vi "Get Buffer Filling Mode.vi"(0 "VISA resource name":refnum<visa-resource-name>, 5 "Buffer Name (defbuffer1)":string="defbuffer1", 11 "error in (no error)":errorcluster) -> (4 "VISA resource name out":refnum<visa-resource-name>, 6 "Data out":string, 15 "error out":errorcluster)   [LabVIEW 2020, in "Keithley 2450.lvlib"]
doc: "This finds whether the reading buffer is filled continuously or is filled once and stops."
uses:
  <instrlib>/Keithley 2450/Keithley 2450.lvlib
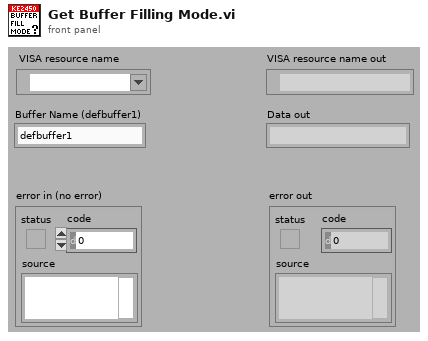
[diagram p1: front panel]
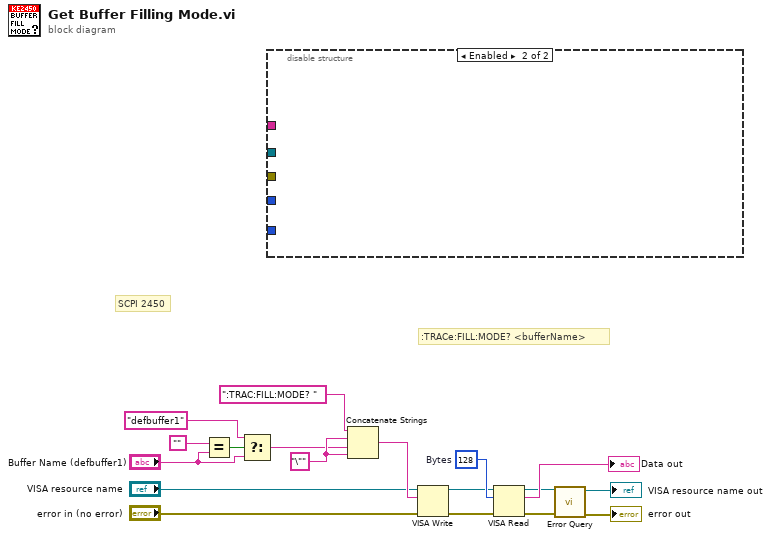
[diagram p0: block diagram]
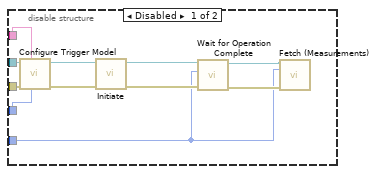
[diagram p2: hidden frame]
diagram:
  w10 = "\""
  w15 = u32 128  # Bytes
  # ":TRACe:FILL:MODE? <bufferName>"
  # "SCPI 2450"
  n1 = Equal?(x="", y="Buffer Name (defbuffer1)") -> (x = y?=w12:bool)
  n2 = Select(t="defbuffer1", s=w12, f="Buffer Name (defbuffer1)") -> (s? t:f=w9:string)
  n3 = disable-structure shown="Enabled" {
    disable-tunnel: _ -> [w25 _]
    disable-tunnel: _ -> [w24 _]
    disable-tunnel: _ -> [w23 _]
    disable-tunnel: _ -> [w22 _]
    disable-tunnel: _ -> [w19 _]
    frame Disabled {
      n4 = call <instrlib>:"Configure Trigger Model.vi"("Trigger Count (1)"=w24, "Buffer Name (defbuffer1)"=w19, "error in (no error)"=w22, "VISA resource name"=w23) -> ("error out"=w20:errorcluster, "VISA resource name out"=w21:refnum<visa-resource-name>)  [unwired: 6 in]
      n5 = call <instrlib>:"Initiate.vi"("error in (no error)"=w20, "VISA resource name"=w21) -> ("error out"=w28:errorcluster, "VISA resource name out"=w29:refnum<visa-resource-name>)  [unwired: 8 out]
      n6 = call <instrlib>:"Wait for Operation Complete.vi"("error in (no error)"=w28, "Timeout (10000 ms)"=w25, "VISA resource name"=w29) -> ("error out"=w27:errorcluster, "VISA resource name out"=w26:refnum<visa-resource-name>)  [unwired: 7 out]
      n7 = call <instrlib>:"Fetch (Measurements).vi"("VISA resource name"=w26, "Timeout (10000 ms)"=w25, "error in (no error)"=w27) -> ()  [unwired: 2 in, 11 out]
    }
    frame Enabled {
    }
  }
  n8 = Concatenate Strings(":TRAC:FILL:MODE? " ("Fetch Measurement"), w10, w9, w10) -> (w16:string)
  n9 = VISA Write(VISA resource name="VISA resource name", write buffer=w16, error in (no error)="error in (no error)") -> (VISA resource name out=w5:refnum<visa-resource-name>, error out=w4:errorcluster)  [unwired: 1 out]
  n10 = VISA Read(VISA resource name=w5, byte count=w15, error in (no error)=w4) -> (VISA resource name out=w3:refnum<visa-resource-name>, read buffer=→"Data out":string, error out=w2:errorcluster)  [unwired: 1 out]
  n11 = call <instrlib>:"Error Query.vi"("error in (no error)"=w2, "VISA resource name"=w3) -> ("error out"=→"error out":errorcluster, "VISA resource name out"=→"VISA resource name out":refnum<visa-resource-name>)  [unwired: 8 out]
